vi "Get Networks.vi"(8 "error in (no error)":errorcluster, 11 "Proto in":refnum<class "Proto.lvclass">) -> (0 "error out":errorcluster, 2 "set":set{set{string}}(c389), 3 "Proto out":refnum<class "Proto.lvclass">)   [LabVIEW 2020, in "Proto.lvclass"]
uses:
  Proto.lvclass
  Proto.lvclass/Proto.ctl
  678eb7b4-9617-4fe5-baf8-81efd0a1ba06.vi
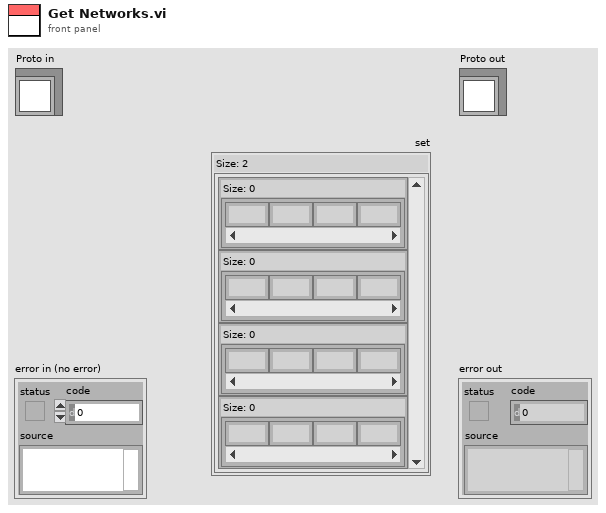
[diagram p1: front panel]
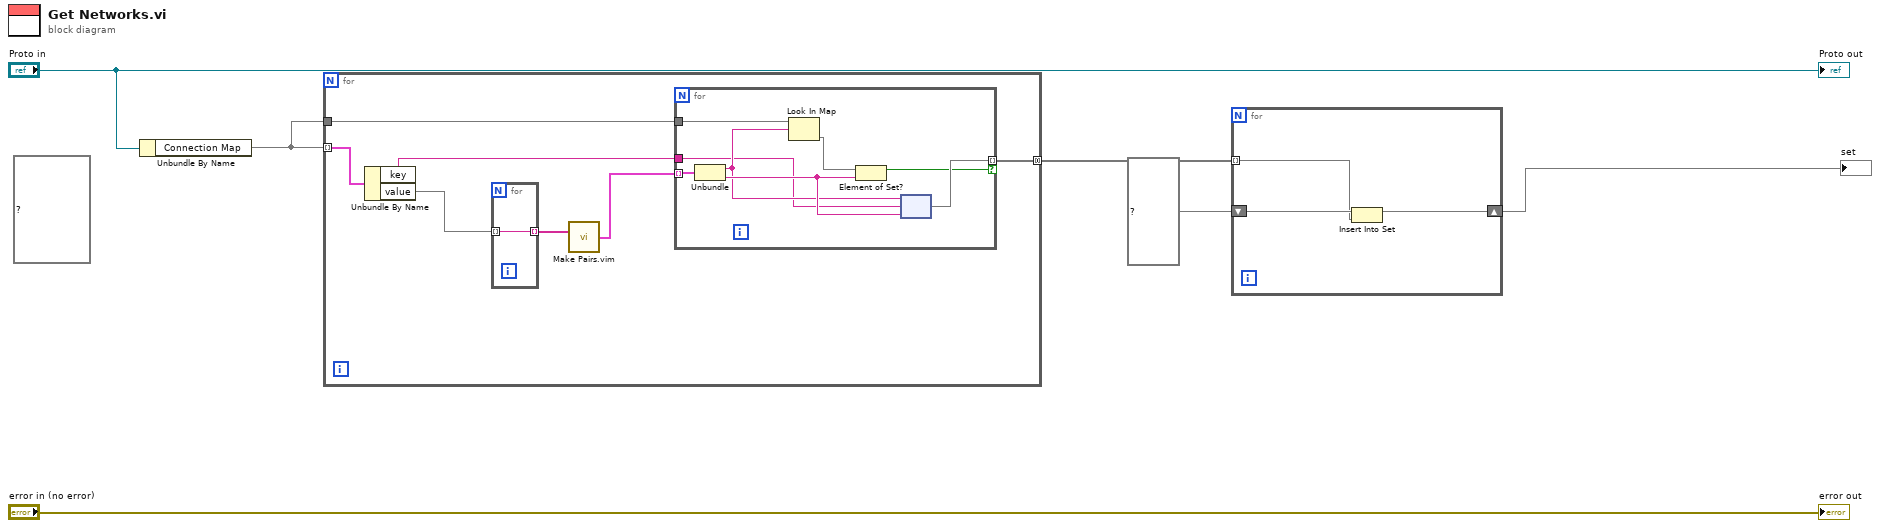
[diagram p0: block diagram]
diagram:
  (unwired) map{string, set{string}} {} ("Connection Map")
  n1 = Unbundle By Name("Proto in") -> ("Connection Map"=w4:map{string, set{string}})
  n2 = for {
    tunnel: w4 -> [w13] mode=indexing
    tunnel: w4 -> [w12]
    tunnel: [w7] -> w1 mode=concatenating
    n3 = Unbundle By Name(w13) -> ("key"=w8:string, "value"=w11:set{string})
    n4 = for {
      tunnel: w11 -> [w22] mode=indexing
      tunnel: [w22] -> w10 mode=indexing
    }
    n5 = call "Make Pairs.vim"("Array"=w10) -> ("Pairs"=w9:cluster{string, string}[])
    n6 = for {
      tunnel: w12 -> [w21]
      tunnel: w9 -> [w20] mode=indexing
      tunnel: w8 -> [w16]
      tunnel: [w15] -> w7 mode=indexing if=w14
      n7 = Unbundle(w20) -> (w17:string, w18:string)
      n8 = Look In Map(map=w21, key=w17) -> (value=w19:set{string})  [unwired: 1 in, 1 out]
      n9 = Element of Set?(10:w18, 11:w19) -> (3:w14:bool)
      n10 = node(w17, w16, w18) -> (w15:set{string})
    }
  }
  n11 = for {
    shift-right: [w24] -> w2
    shift-left: set{set{string}} {} ("set") -> [w25]
    tunnel: w1 -> [w23] mode=indexing
    n12 = Insert Into Set(10:w23, 11:w25) -> (3:w24:set{set{string}})  [unwired: 1 out]
  }
  "set" <- w2
  "error out" <- "error in (no error)"
  "Proto out" <- "Proto in"
